vi "Timer_TestPanel.vi"() -> ()   [LabVIEW 2024]
doc: "Test Panel for Demonstrating Two Independent Timers Utilizing DVRs.\n\n--------\nPaulo Rossi\nprossi@aurumautomation.ca\n©2024 Aurum Automation Inc.\nOpen-Sourced per GNU GPL v3\n\nYou should have received a copy of the GNU General Public License along with this program. If not, see <https://www.gnu.org/licenses/>."
panel:
  out "Time Elapsed (s) 2":dbl
  out "Is Time Elapsed? 2":bool
  in  "Reset Timer 2":bool
  in  "Stop Timer 2":bool
  in  "error in (no error) 2":errorcluster
  out "error out 2":errorcluster
  in  "Target Time (s) 2":dbl=15.0 format="%#_13g"
  in  "Target Time (s)":dbl=15.0 format="%#_13g"
  in  "Stop Timer":bool
  in  "Reset Timer":bool
  out "error out":errorcluster
  out "Is Time Elapsed?":bool
  out "Time Elapsed (s)":dbl
  in  "error in (no error)":errorcluster
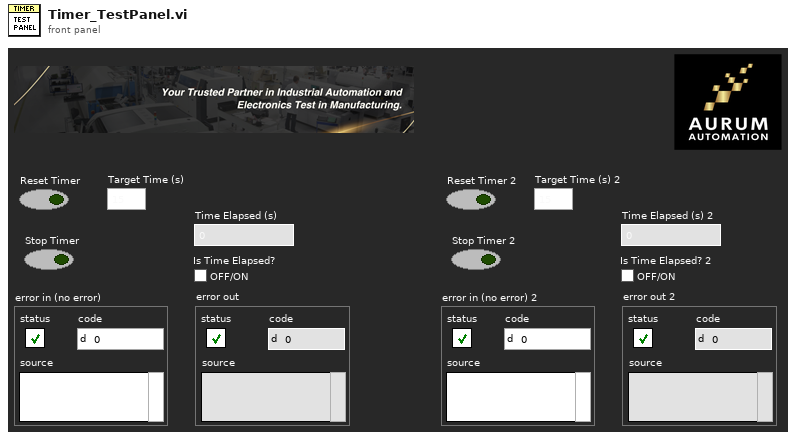
[diagram p1: front panel]
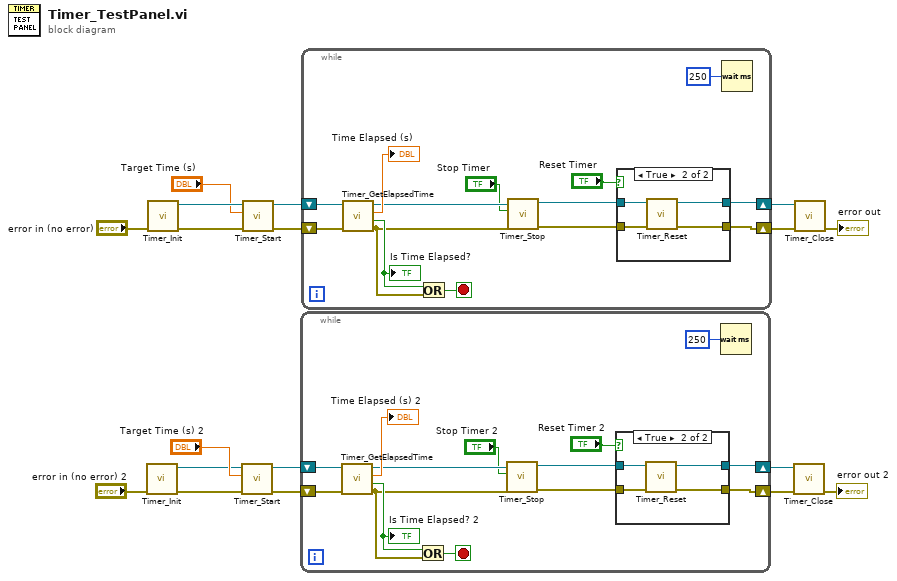
[diagram p0: block diagram]
diagram:
  n1 = call "Timer_Init.vi"("error in (no error)"="error in (no error) 2") -> ("error out"=w2:errorcluster, "Timer Data Reference (out)"=w3:refnum<data-value>)  [unwired: 9 in]
  n2 = call "Timer_Init.vi"("error in (no error)"="error in (no error)") -> ("error out"=w17:errorcluster, "Timer Data Reference (out)"=w16:refnum<data-value>)  [unwired: 9 in]
  n3 = call "Timer_Start.vi"("error in (no error)"=w2, "Target Time (s)"="Target Time (s) 2", "Timer Data Reference (in)"=w3) -> ("error out"=w5:errorcluster, "Timer Data Reference (out)"=w6:refnum<data-value>)  [unwired: 7 in]
  n4 = call "Timer_Start.vi"("error in (no error)"=w17, "Target Time (s)"="Target Time (s)", "Timer Data Reference (in)"=w16) -> ("error out"=w14:errorcluster, "Timer Data Reference (out)"=w13:refnum<data-value>)  [unwired: 7 in]
  n5 = while {
    shift-right: [w22] -> w7
    shift-left: w5 -> [w30]
    shift-right: [w21] -> w8
    shift-left: w6 -> [w29]
    stop <- w31 stop-if-true
    n6 = call "Timer_GetElapsedTime.vi"("error in (no error)"=w30, "Timer Data Reference (in)"=w29) -> ("error out"=w25:errorcluster, "Is Time Elapsed?"=w27:bool, "Time Elapsed (s)"=→"Time Elapsed (s) 2":dbl, "Timer Data Reference (out)"=w26:refnum<data-value>)  [unwired: 6 in]
    "Is Time Elapsed? 2" <- w27
    n7 = Or(x=w27, y=w25) -> (x .or. y?=w31:bool)
    n8 = call "Timer_Stop.vi"("error in (no error)"=w25, "Is Paused?"="Stop Timer 2", "Timer Data Reference (in)"=w26) -> ("error out"=w23:errorcluster, "Timer Data Reference (out)"=w24:refnum<data-value>)  [unwired: 7 in]
    n9 = case shown="True" "Reset Timer 2" {
      tunnel: w24 -> [w34 w38]
      tunnel: w23 -> [w33 w37]
      tunnel: [w33 w36] -> w22
      tunnel: [w34 w35] -> w21
      frame False {
      }
      frame True {
        n10 = call "Timer_Reset.vi"("error in (no error)"=w37, "Timer Data Reference (in)"=w38) -> ("error out"=w36:errorcluster, "Timer Data Reference (out)"=w35:refnum<data-value>)  [unwired: 8 in]
      }
    }
    n11 = Wait (ms)(milliseconds to wait=u32 250) -> ()  [unwired: 1 out]
  }
  n12 = while {
    shift-right: [w42] -> w12
    shift-left: w14 -> [w50]
    shift-right: [w41] -> w11
    shift-left: w13 -> [w49]
    stop <- w51 stop-if-true
    n13 = call "Timer_GetElapsedTime.vi"("error in (no error)"=w50, "Timer Data Reference (in)"=w49) -> ("error out"=w45:errorcluster, "Is Time Elapsed?"=w47:bool, "Time Elapsed (s)"=→"Time Elapsed (s)":dbl, "Timer Data Reference (out)"=w46:refnum<data-value>)  [unwired: 6 in]
    "Is Time Elapsed?" <- w47
    n14 = Or(x=w47, y=w45) -> (x .or. y?=w51:bool)
    n15 = call "Timer_Stop.vi"("error in (no error)"=w45, "Is Paused?"="Stop Timer", "Timer Data Reference (in)"=w46) -> ("error out"=w43:errorcluster, "Timer Data Reference (out)"=w44:refnum<data-value>)  [unwired: 7 in]
    n16 = case shown="True" "Reset Timer" {
      tunnel: w44 -> [w54 w58]
      tunnel: w43 -> [w53 w57]
      tunnel: [w53 w56] -> w42
      tunnel: [w54 w55] -> w41
      frame False {
      }
      frame True {
        n17 = call "Timer_Reset.vi"("error in (no error)"=w57, "Timer Data Reference (in)"=w58) -> ("error out"=w56:errorcluster, "Timer Data Reference (out)"=w55:refnum<data-value>)  [unwired: 8 in]
      }
    }
    n18 = Wait (ms)(milliseconds to wait=u32 250) -> ()  [unwired: 1 out]
  }
  n19 = call "Timer_Close.vi"("error in (no error)"=w7, "Timer Data Reference (in)"=w8) -> ("error out"=→"error out 2":errorcluster)  [unwired: 9 in]
  n20 = call "Timer_Close.vi"("error in (no error)"=w12, "Timer Data Reference (in)"=w11) -> ("error out"=→"error out":errorcluster)  [unwired: 9 in]
